vi "z-function-filter.vi"(8 "error in (no error)":errorcluster, 10 "z-Points IN":dbl[](array[numeric]), 11 "TrajectoryAK101022Resonance in":refnum<class "TrajectoryAK101022Resonance.lvclass">) -> (0 "error out":errorcluster, 2 "z-Points OUT":dbl[](array[numeric]), 3 "TrajectoryAK101022Resonance out":refnum<class "TrajectoryAK101022Resonance.lvclass">)   [LabVIEW 2010, in "TrajectoryAK101022Resonance.lvclass"]
uses:
  TrajectoryAK101022Resonance.lvclass
  TrajectoryAK101022Resonance.lvclass/TrajectoryAK101022Resonance.ctl
  <vilib>/ptbypt/NI_PtbyPt.lvlib
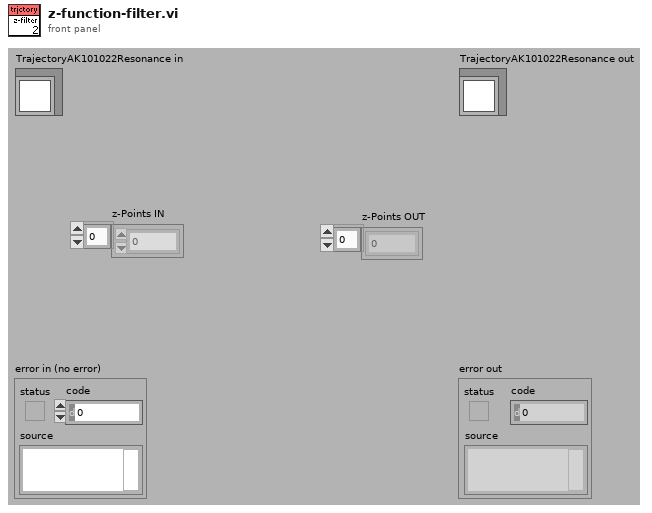
[diagram p1: front panel]
types:
  T1 = enum16{"Lowpass", "Highpass", "Bandpass", "Bandstop"}
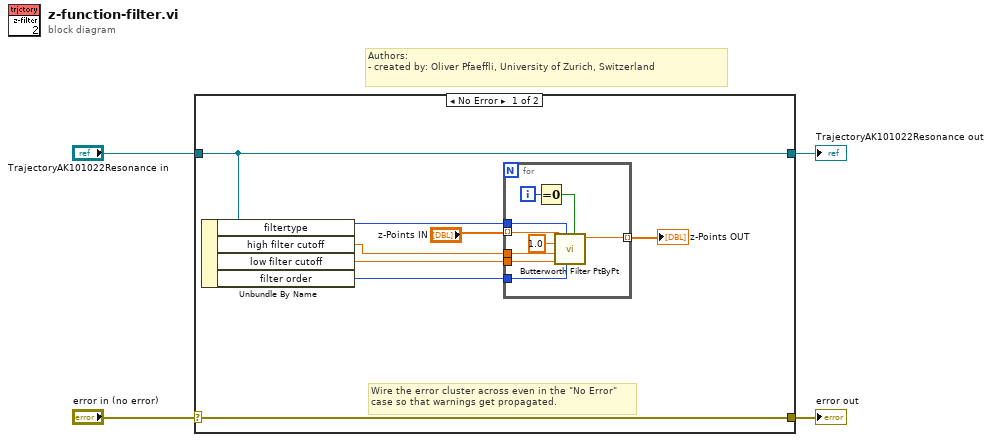
[diagram p0: block diagram]
diagram:
  # "Authors: \n- created by: Oliver Pfaeffli, University of Zurich, Switzerland"
  n1 = case shown="No Error" "error in (no error)" {
    selector: "error in (no error)" -> [w12 w23]
    tunnel: [w12 w23] -> w3
    tunnel: [w11 w22] -> w1
    tunnel: "TrajectoryAK101022Resonance in" -> [w11 w22]
    frame No Error {
      # "Wire the error cluster across even in the \"No Error\"\ncase so that warnings get propagated."
      n2 = Unbundle By Name(w11) -> ("filtertype"=w10:T1, "high filter cutoff"=w9:dbl, "low filter cutoff"=w8:dbl, "filter order"=w7:u16)
      n3 = for {
        tunnel: w10 -> [w21]
        tunnel: w9 -> [w20]
        tunnel: w8 -> [w19]
        tunnel: w7 -> [w18]
        tunnel: "z-Points IN" -> [w16] mode=indexing
        tunnel: [w15] -> w5 mode=indexing
        i -> [w14]
        n4 = Equal To 0?(x=w14) -> (x = 0?=w13:bool)
        n5 = call <vilib>:"Butterworth Filter PtByPt.vi"("initialize"=w13, "order"=w18, "filter type"=w21, "low cutoff freq: fl"=w19, "high cutoff freq: fh"=w20, "sampling freq: fs"=1.0, "x"=w16) -> ("Filtered x"=w15:dbl)  [unwired: 2 in, 1 out]
      }
      "z-Points OUT" <- w5
    }
    frame Error {
    }
  }
  "error out" <- w3
  "TrajectoryAK101022Resonance out" <- w1
